vi "Configure.vi"(8 "error in (no error)":errorcluster, 9 "Default Path":path, 10 "Interactive?":bool, 11 "Report Generator in":refnum<class "Report Generator.lvclass">) -> (0 "error out":errorcluster, 3 "Report Generator out":refnum<class "Report Generator.lvclass">)   [LabVIEW 2020, in "Report Generation.lvlib" / "Report Generator.lvclass"]
uses:
  Report Generator.lvclass
  Report Generator.lvclass/Report Generator.ctl
  User Interface/Process/Process.lvclass
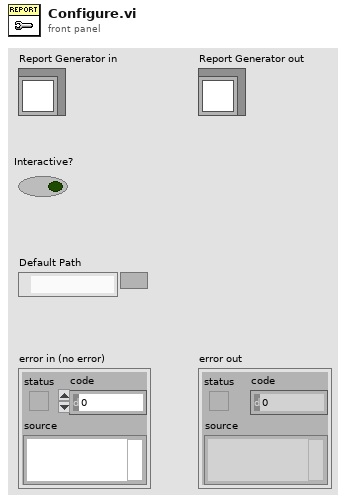
[diagram p1: front panel]
types:
  T1 = cluster{"Interactive?":bool, "Default Path":path}
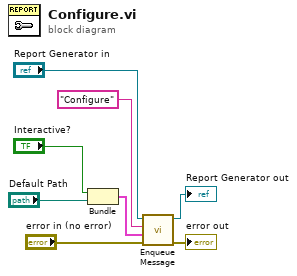
[diagram p0: block diagram]
diagram:
  n1 = Bundle("Interactive?"="Interactive?", "Default Path"="Default Path") -> (w1:T1)  [unwired: 1 in]
  n2 = call "Enqueue Message.vi"("error in (no error)"="error in (no error)", "Message Data"=w1, "Message"="Configure", "Process In"="Report Generator in") -> ("error out"=→"error out":errorcluster, "Process Out"=→"Report Generator out":refnum<class "Report Generator.lvclass">)  [unwired: 6 in]
